vi "weblab-1.vi"() -> ()   [LabVIEW 2011]
panel:
  out "Waveform Chart":dbl[](graph)
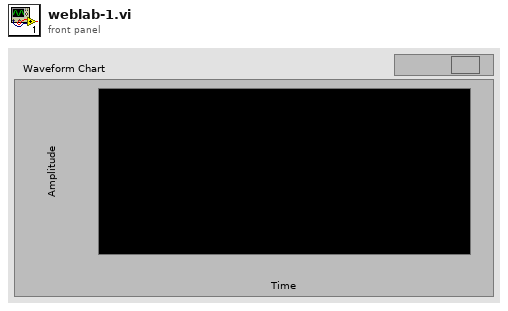
[diagram p1: front panel]
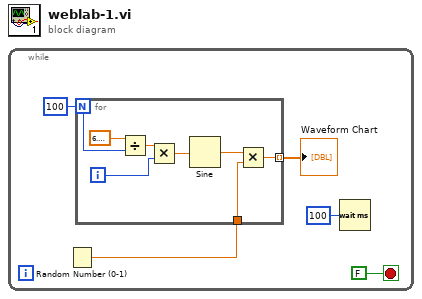
[diagram p0: block diagram]
diagram:
  n1 = while {
    stop <- FALSE stop-if-true
    n2 = Random Number (0-1)() -> (number: 0 to 1=w4:dbl)
    n3 = for {
      N: 100 -> [w12]
      tunnel: [w8] -> w2 mode=indexing
      tunnel: w4 -> [w6]
      i -> [w10]
      n4 = Divide(x=6.283185307179586, y=w12) -> (x/y=w11:dbl)
      n5 = Multiply(x=w11, y=w10) -> (x*y=w9:dbl)
      n6 = Sine(x=w9) -> (sin(x)=w7:dbl)
      n7 = Multiply(x=w7, y=w6) -> (x*y=w8:dbl)
    }
    "Waveform Chart" <- w2
    n8 = Wait (ms)(milliseconds to wait=u32 100) -> ()  [unwired: 1 out]
  }
